vi "test.vi"() -> ()   [LabVIEW 2016]
panel:
  in  "M1DO0 R5 inf":bool
  out "M3AI0 R5 pH":dbl
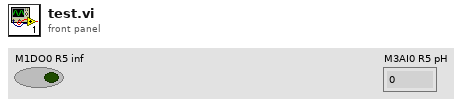
[diagram p1: front panel]
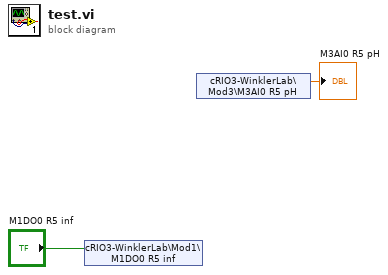
[diagram p0: block diagram]
diagram:
  n1 = shared-variable "cRIO3-WinklerLab\\Mod1\\M1DO0 R5 inf"("M1DO0 R5 inf") -> ()  [unwired: 1 in, 1 out]
  n2 = shared-variable "cRIO3-WinklerLab\\Mod3\\M3AI0 R5 pH"() -> (→"M3AI0 R5 pH":dbl)  [unwired: 1 in, 1 out]
